vi "PCO_Convert16TO8.vi"(0 "ph":u64, 1 "height":i32, 5 "mode":i32, 7 "icolmode":i32, 9 "width":i32, 11 "error in (no error)":errorcluster {"code" format="%x"}, 12 "b16":u16[][](array[numeric])=array1x4097[4097 elements]) -> (4 "ph out":u64, 6 "ErrorMessage":i32 format="%x", 8 "b8":u8[][](array[numeric]), 15 "error out":errorcluster {"code" format="%x"})   [LabVIEW 2020, in "Convert.lvlib"]
doc: "int PCOCONVERT_API PCO_Convert16TO8(HANDLE ph, int mode, int icolmode, int width,int height, word *b16, byte *b8);"
uses:
  Convert.lvlib
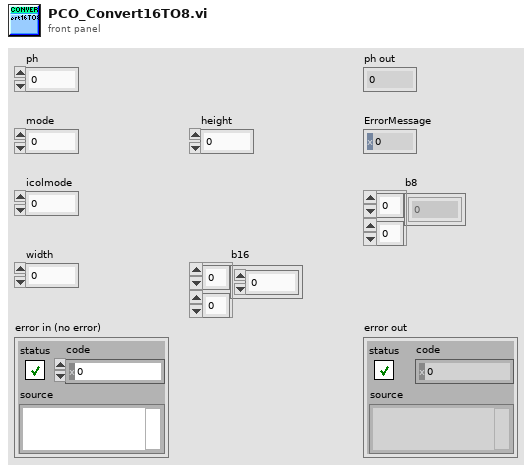
[diagram p1: front panel]
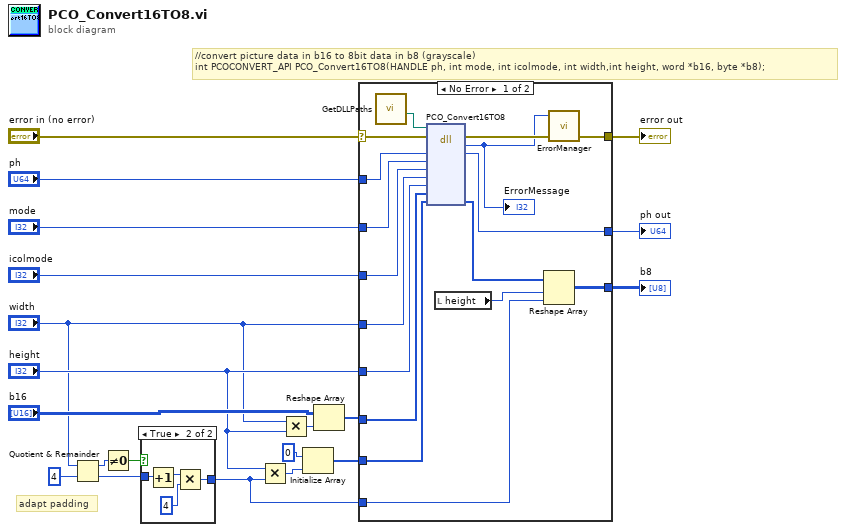
[diagram p0: block diagram]
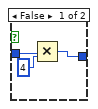
[diagram p2: hidden frame]
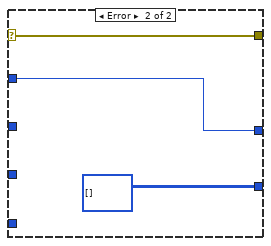
[diagram p3: hidden frame]
diagram:
  # "adapt padding"
  # "//convert picture data in b16 to 8bit data in b8 (grayscale)\nint PCOCONVERT_API PCO_Convert16TO8(HANDLE ph, int mode, int icolmode, int width,int height, word *b16, byte *b8);"
  n1 = Quotient & Remainder(x="width", y=4) -> (x-y*floor(x/y)=w4:i32, floor(x/y)=w2:i32)
  n2 = Not Equal To 0?(x=w4) -> (x != 0?=w3:bool)
  n3 = case shown="True" w3 {
    tunnel: w2 -> [w23 w27]
    tunnel: [w21 w24] -> w1
    frame False {
      n4 = Multiply(x=w23, y=4) -> (x*y=w21:i32)
    }
    frame True {
      n5 = Increment(x=w27) -> (x+1=w25:i32)
      n6 = Multiply(x=w25, y=4) -> (x*y=w24:i32)
    }
  }
  n7 = Multiply(x="height", y=w1) -> (x*y=w14:i32)
  n8 = Multiply(x="width", y="height") -> (x*y=w11:i32)
  n9 = Initialize Array(u8 0 ("element"), w14) -> (w16:u8[])
  n10 = Reshape Array("b16", w11) -> (w10:u16[])
  n11 = case shown="No Error" "error in (no error)" {
    selector: "error in (no error)" -> [w36 w47]
    tunnel: "ph" -> [w44 w46]
    tunnel: [w43 w46] -> w19
    tunnel: "mode" -> [w42 _]
    tunnel: "icolmode" -> [w41 _]
    tunnel: w10 -> [w40 _]
    tunnel: w16 -> [w39 _]
    tunnel: [w29 u8[][] [] ("b8")] -> w7
    tunnel: [w35 w47] -> w15
    tunnel: "width" -> [w38 _]
    tunnel: "height" -> [w37 _]
    tunnel: w1 -> [w28 _]
    frame No Error {
      n12 = call "GetDLLPaths.vi"() -> ("PCO_Conv_Path"=w32:path)  [unwired: 9 in, 2 out]
      n13 = dll-call lib="?" fn="PCO_Convert16TO8"(path in=w32, error in=w36, "ph"=w44, "mode"=w42, "icolmode"=w41, "width"=w38, "height"=w37, "b16"=w40, "b8"=w39) -> (error out=w34:errorcluster, "return type"=w33:i32, "ph"=w43:u64, "b8"=w31:u8[])  [unwired: 6 in, 1 out]
      "ErrorMessage" <- w33
      n14 = local read "height"() -> (w30:i32)
      n15 = Reshape Array(w31, w30, w28) -> (w29:u8[][])
      n16 = call "ErrorManager.vi"("error in (no error)"=w34, "error code"=w33) -> ("error out"=w35:errorcluster)  [unwired: 3 in]
    }
    frame Error {
    }
  }
  "ph out" <- w19
  "b8" <- w7
  "error out" <- w15
